vi "getAcquisitionSettings.vi"(8 "error in (no error)":errorcluster, 11 "AndorIKonAcquisitor in":refnum<class "AndorIKonAcquisitor.lvclass">) -> (0 "error out":errorcluster, 3 "AndorIKonAcquisitor out":refnum<class "AndorIKonAcquisitor.lvclass">)   [LabVIEW 2011, in "Hardware.lvlib" / "Channels.lvlib" / "AndorIKonAcquisitor.lvclass"]
uses:
  AndorIKonAcquisitor.lvclass
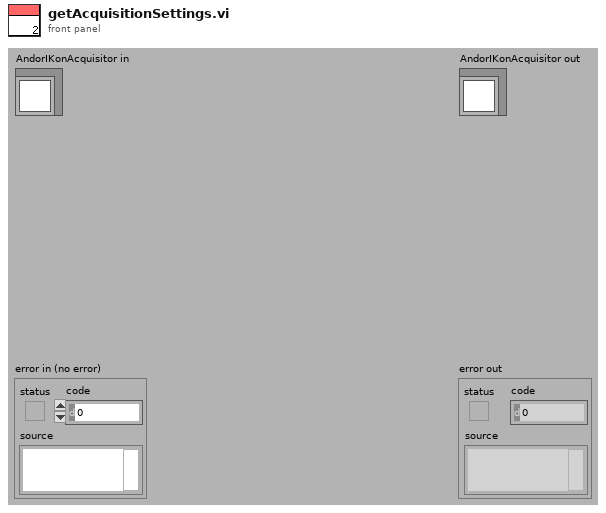
[diagram p1: front panel]
types:
  T1 = cluster{"Acquisition mode":dbl, "Readout Mode":dbl, "Gain":dbl}
  T2 = cluster{"shutter Open Time":dbl, "Shutter Close Time":dbl, "Exposure Time":dbl, " AccumulatedCycleTime":dbl, " KineticCycleTime":dbl, "Number of Accumulations":dbl, "Number in Kinetic Series ":dbl, "Shutter Mode":dbl}
  T3 = cluster{"Exposure Time":dbl, "Accumulation Cycle Time":dbl, " Kinetic Cycle Time":dbl}
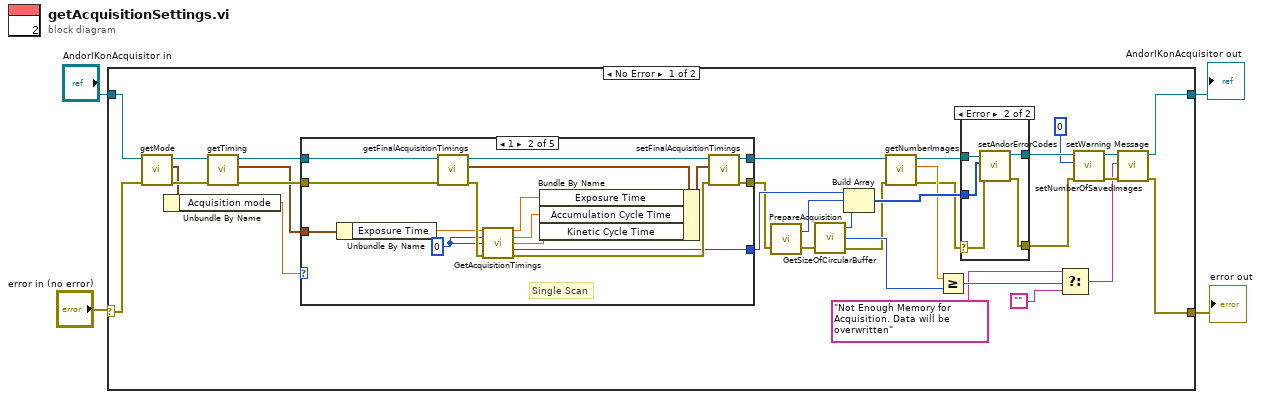
[diagram p0: block diagram]
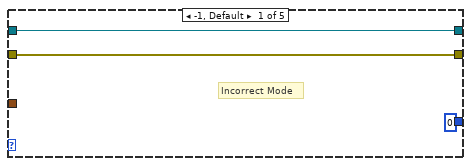
[diagram p3: hidden frame]
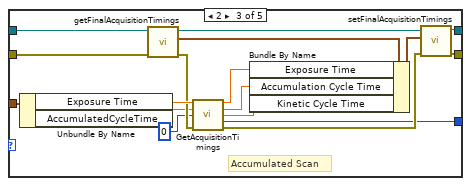
[diagram p4: hidden frame]
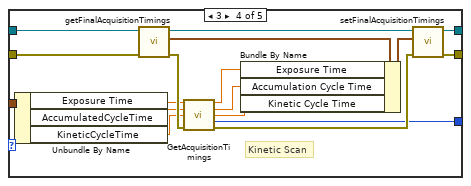
[diagram p5: hidden frame]
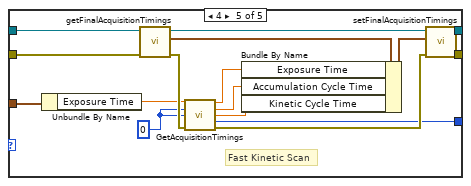
[diagram p6: hidden frame]
diagram:
  n1 = case shown="No Error" "error in (no error)" {
    selector: "error in (no error)" -> [w36 w114]
    tunnel: [w6 w114] -> w3
    tunnel: [w5 w113] -> w1
    tunnel: "AndorIKonAcquisitor in" -> [w35 w113]
    frame No Error {
      n2 = call-dynamic "getMode.vi"("error in (no error)"=w36, "CameraAcquisitor.lvclass in"=w35) -> ("error out"=w33:errorcluster, "Mode"=w32:T1, "CameraAcquisitor.lvclass out"=w34:refnum<class "AndorIKonAcquisitor.lvclass">)  [unwired: 7 in]
      n3 = Unbundle By Name(w32) -> ("Acquisition mode"=w31:dbl)
      n4 = call-dynamic "getTiming.vi"("error in (no error)"=w33, "CameraAcquisitor.lvclass in"=w34) -> ("error out"=w29:errorcluster, "Timing"=w28:T2, "CameraAcquisitor.lvclass out"=w30:refnum<class "AndorIKonAcquisitor.lvclass">)  [unwired: 7 in]
      n5 = case shown="1" w31 {
        tunnel: w28 -> [_ w62 w68 w83 w101]
        tunnel: w30 -> [w45 w53 w70 w87 w103]
        tunnel: w29 -> [w44 w51 w69 w86 w102]
        tunnel: [w45 w50 w66 w84 w100] -> w18
        tunnel: [w44 w49 w67 w85 w97] -> w25
        tunnel: [0 w48 w64 w80 w99] -> w26
        frame -1, Default {
          # "Incorrect Mode"
        }
        frame 1 {
          w47 = 0
          # "Single Scan"
          n6 = Unbundle By Name(w62) -> ("Exposure Time"=w52:dbl)
          n7 = call-dynamic "getFinalAcquisitionTimings.vi"("error in (no error)"=w51, "CameraAcquisitor.lvclass in"=w53) -> ("error out"=w61:errorcluster, "Final Acquisition Timings"=w58:T3, "CameraAcquisitor.lvclass out"=w60:refnum<class "AndorIKonAcquisitor.lvclass">)  [unwired: 7 in]
          n8 = call <userlib>:"GetAcquisitionTimings.vi"("exposure input"=w52, "accumulate input"=w47, "kinetic input"=w47, "error in (no error)"=w61) -> ("exposure"=w55:sgl, "accumulate"=w56:sgl, "kinetic"=w57:sgl, "DLL error code"=w48:u32, "error out"=w54:errorcluster)  [unwired: 7 in]
          n9 = Bundle By Name(cluster=w58, "Exposure Time"=w55, "Accumulation Cycle Time"=w56, "Kinetic Cycle Time"=w57) -> (w59:T3)
          n10 = call-dynamic "setFinalAcquisitionTimings.vi"("error in (no error)"=w54, "Final Acquisition Timings"=w59, "CameraAcquisitor.lvclass in"=w60) -> ("error out"=w49:errorcluster, "CameraAcquisitor.lvclass out"=w50:refnum<class "AndorIKonAcquisitor.lvclass">)  [unwired: 7 in]
        }
        frame 2 {
          # "Accumulated Scan"
          n11 = Unbundle By Name(w68) -> ("Exposure Time"=w79:dbl, "AccumulatedCycleTime"=w65:dbl)
          n12 = call-dynamic "getFinalAcquisitionTimings.vi"("error in (no error)"=w69, "CameraAcquisitor.lvclass in"=w70) -> ("error out"=w71:errorcluster, "Final Acquisition Timings"=w74:T3, "CameraAcquisitor.lvclass out"=w72:refnum<class "AndorIKonAcquisitor.lvclass">)  [unwired: 7 in]
          n13 = call <userlib>:"GetAcquisitionTimings.vi"("exposure input"=w79, "accumulate input"=w65, "kinetic input"=0, "error in (no error)"=w71) -> ("exposure"=w77:sgl, "accumulate"=w76:sgl, "kinetic"=w75:sgl, "DLL error code"=w64:u32, "error out"=w78:errorcluster)  [unwired: 7 in]
          n14 = Bundle By Name(cluster=w74, "Exposure Time"=w77, "Accumulation Cycle Time"=w76, "Kinetic Cycle Time"=w75) -> (w73:T3)
          n15 = call-dynamic "setFinalAcquisitionTimings.vi"("error in (no error)"=w78, "Final Acquisition Timings"=w73, "CameraAcquisitor.lvclass in"=w72) -> ("error out"=w67:errorcluster, "CameraAcquisitor.lvclass out"=w66:refnum<class "AndorIKonAcquisitor.lvclass">)  [unwired: 7 in]
        }
        frame 3 {
          # "Kinetic Scan"
          n16 = Unbundle By Name(w83) -> ("Exposure Time"=w88:dbl, "AccumulatedCycleTime"=w82:dbl, "KineticCycleTime"=w81:dbl)
          n17 = call-dynamic "getFinalAcquisitionTimings.vi"("error in (no error)"=w86, "CameraAcquisitor.lvclass in"=w87) -> ("error out"=w96:errorcluster, "Final Acquisition Timings"=w93:T3, "CameraAcquisitor.lvclass out"=w95:refnum<class "AndorIKonAcquisitor.lvclass">)  [unwired: 7 in]
          n18 = call <userlib>:"GetAcquisitionTimings.vi"("exposure input"=w88, "accumulate input"=w82, "kinetic input"=w81, "error in (no error)"=w96) -> ("exposure"=w90:sgl, "accumulate"=w91:sgl, "kinetic"=w92:sgl, "DLL error code"=w80:u32, "error out"=w89:errorcluster)  [unwired: 7 in]
          n19 = Bundle By Name(cluster=w93, "Exposure Time"=w90, "Accumulation Cycle Time"=w91, "Kinetic Cycle Time"=w92) -> (w94:T3)
          n20 = call-dynamic "setFinalAcquisitionTimings.vi"("error in (no error)"=w89, "Final Acquisition Timings"=w94, "CameraAcquisitor.lvclass in"=w95) -> ("error out"=w85:errorcluster, "CameraAcquisitor.lvclass out"=w84:refnum<class "AndorIKonAcquisitor.lvclass">)  [unwired: 7 in]
        }
        frame 4 {
          w98 = 0
          # "Fast Kinetic Scan"
          n21 = Unbundle By Name(w101) -> ("Exposure Time"=w104:dbl)
          n22 = call-dynamic "getFinalAcquisitionTimings.vi"("error in (no error)"=w102, "CameraAcquisitor.lvclass in"=w103) -> ("error out"=w112:errorcluster, "Final Acquisition Timings"=w109:T3, "CameraAcquisitor.lvclass out"=w111:refnum<class "AndorIKonAcquisitor.lvclass">)  [unwired: 7 in]
          n23 = call <userlib>:"GetAcquisitionTimings.vi"("exposure input"=w104, "accumulate input"=w98, "kinetic input"=w98, "error in (no error)"=w112) -> ("exposure"=w106:sgl, "accumulate"=w107:sgl, "kinetic"=w108:sgl, "DLL error code"=w99:u32, "error out"=w105:errorcluster)  [unwired: 7 in]
          n24 = Bundle By Name(cluster=w109, "Exposure Time"=w106, "Accumulation Cycle Time"=w107, "Kinetic Cycle Time"=w108) -> (w110:T3)
          n25 = call-dynamic "setFinalAcquisitionTimings.vi"("error in (no error)"=w105, "Final Acquisition Timings"=w110, "CameraAcquisitor.lvclass in"=w111) -> ("error out"=w97:errorcluster, "CameraAcquisitor.lvclass out"=w100:refnum<class "AndorIKonAcquisitor.lvclass">)  [unwired: 7 in]
        }
      }
      n26 = call <userlib>:"PrepareAcquisition.vi"("error in (no error)"=w25) -> ("error out"=w20:errorcluster, "DLL error code"=w24:u32)  [unwired: 1 in]
      n27 = call <userlib>:"GetSizeOfCircularBuffer.vi"("error in (no error)"=w20) -> ("error out"=w14:errorcluster, "index"=w15:u32, "DLL error code"=w19:u32)  [unwired: 2 in]
      n28 = Build Array(w26, w24, w19) -> (w27:u32[])
      n29 = call-dynamic "getNumberImages.vi"("error in (no error)"=w14, "CameraAcquisitor.lvclass in"=w18) -> ("error out"=w13:errorcluster, "Number of Images"=w16:dbl, "CameraAcquisitor.lvclass out"=w17:refnum<class "AndorIKonAcquisitor.lvclass">)  [unwired: 7 in]
      n30 = Greater Or Equal?(x=w16, y=w15) -> (x >= y?=w12:bool)
      n31 = case shown="Error" w13 {
        selector: w13 -> [w38 w40]
        tunnel: w17 -> [w37 w43]
        tunnel: [w37 w41] -> w23
        tunnel: [w38 w42] -> w21
        tunnel: w27 -> [_ w39]
        frame No Error {
        }
        frame Error {
          n32 = call-dynamic "setAndorErrorCodes.vi"("error in (no error)"=w40, "Andor Error Codes"=w39, "AndorIKonAcquisitor.lvclass in"=w43) -> ("error out"=w42:errorcluster, "AndorIKonAcquisitor.lvclass out"=w41:refnum<class "AndorIKonAcquisitor.lvclass">)  [unwired: 7 in]
        }
      }
      n33 = Select(t="Not Enough Memory for Acquisition. Data will be overwritten", s=w12, f="") -> (s? t:f=w7:string)
      n34 = call "setNumberOfSavedImages.vi"("error in (no error)"=w21, "NumberOfSavedImages"=0, "AndorIKonAcquisitor.lvclass in"=w23) -> ("error out"=w8:errorcluster, "AndorIKonAcquisitor.lvclass out"=w9:refnum<class "AndorIKonAcquisitor.lvclass">)  [unwired: 7 in]
      n35 = call-dynamic "setWarning Message.vi"("error in (no error)"=w8, "Warning Message"=w7, "CameraAcquisitor.lvclass in"=w9) -> ("error out"=w6:errorcluster, "CameraAcquisitor.lvclass out"=w5:refnum<class "AndorIKonAcquisitor.lvclass">)  [unwired: 7 in]
    }
    frame Error {
    }
  }
  "error out" <- w3
  "AndorIKonAcquisitor out" <- w1
